vi "svl_Exp Avg Resampled Level Core (N Ch).vi"(0 "scaled signals":T1(array[cluster]) {"even angle signal" format="%.2f"; "dr" format="%.2f"; "r0" format="%.2f"}, 2 "sampling frequency [Hz]":dbl, 5 "filter coefficients (in)":T2 {"Forward Coefficients" format="%.2f"; "Reverse Coefficients" format="%.2f"}, 7 "initial values (impulse)":dbl[](array[numeric]) format="%.2f", 9 "init/cont (init:F)":bool, 11 "error in (no error)":errorcluster, 12 "initial values (exp)":dbl[](array[numeric]) format="%.2f", 13 "exponential mode":enum16{"Slow", "Fast", "Impulse", "Custom"}(ring)=enum."Fast") -> (4 "exp avg signals":T1(array[cluster]) {"even angle signal" format="%.2f"; "dr" format="%.2f"; "r0" format="%.2f"}, 6 "dup filter coefficients":T2 {"Forward Coefficients" format="%.2f"; "Reverse Coefficients" format="%.2f"}, 8 "final values (impulse)":dbl[](array[numeric]) format="%.2f", 14 "final values (exp)":dbl[](array[numeric]) format="%.2f", 15 "error out":errorcluster)   [LabVIEW 2017]
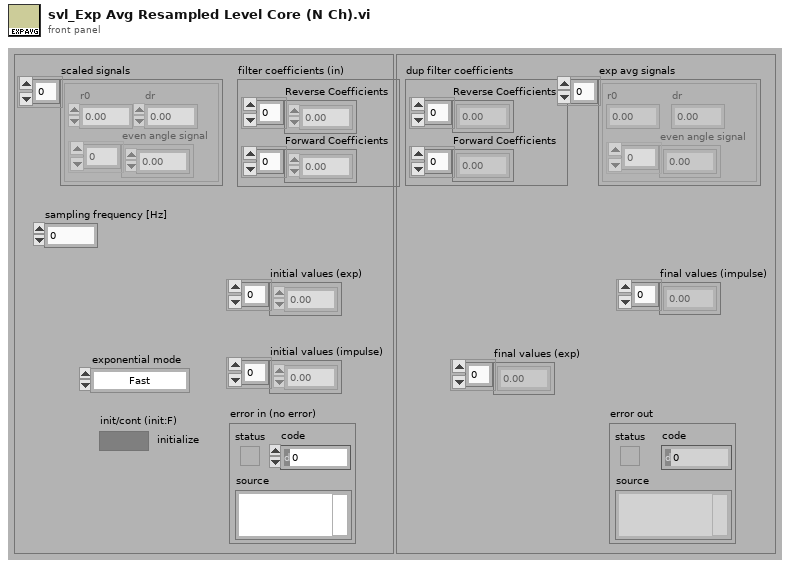
[diagram p1: front panel]
types:
  T1 = cluster{"r0":dbl, "dr":dbl, "even angle signal":dbl[]}[]
  T2 = cluster{"Reverse Coefficients":dbl[], "Forward Coefficients":dbl[]}
  T3 = cluster{"r0":dbl, "dr":dbl, "even angle signal":dbl[]}
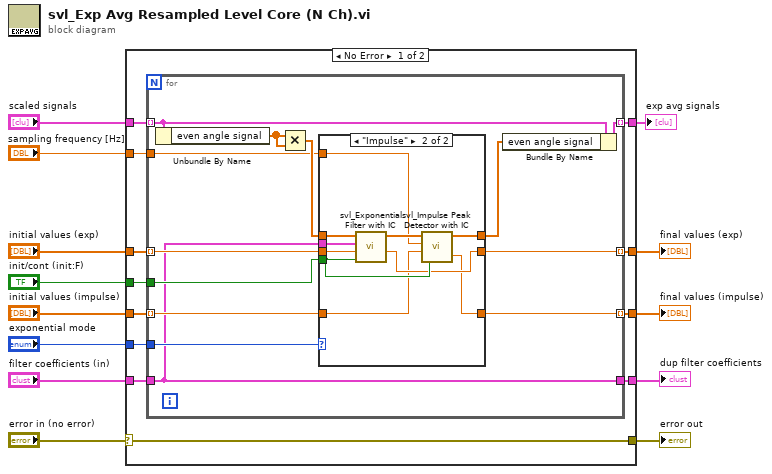
[diagram p0: block diagram]
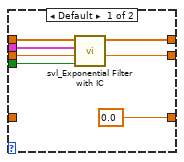
[diagram p2: hidden frame]
diagram:
  n1 = case shown="No Error" "error in (no error)" {
    selector: "error in (no error)" -> [w19 w57]
    tunnel: "initial values (exp)" -> [w25 w59]
    tunnel: "scaled signals" -> [w24 w56]
    tunnel: "exponential mode" -> [w23 _]
    tunnel: "filter coefficients (in)" -> [w22 w58]
    tunnel: "init/cont (init:F)" -> [w21 _]
    tunnel: [w20 w59] -> w8
    tunnel: [w19 w57] -> w7
    tunnel: "initial values (impulse)" -> [w18 w60]
    tunnel: [w17 w60] -> w5
    tunnel: [w16 w58] -> w4
    tunnel: "sampling frequency [Hz]" -> [w15 _]
    tunnel: [w14 w56] -> w1
    frame No Error {
      n2 = for {
        tunnel: w24 -> [w29] mode=indexing
        tunnel: w25 -> [w36] mode=indexing
        tunnel: w23 -> [w38]
        tunnel: w22 -> [w31]
        tunnel: w21 -> [w35]
        tunnel: [w34] -> w20 mode=indexing
        tunnel: w18 -> [w33] mode=indexing
        tunnel: [w32] -> w17 mode=indexing
        tunnel: [w31] -> w16
        tunnel: w15 -> [w30]
        tunnel: [w28] -> w14 mode=indexing
        n3 = Unbundle By Name(w29) -> ("even angle signal"=w26:dbl[])
        n4 = Multiply(x=w26, y=w26) -> (x*y=w37:dbl[])
        n5 = case shown="\"Impulse\"" w38 {
          tunnel: w37 -> [w45 w55]
          tunnel: w31 -> [w44 w54]
          tunnel: w36 -> [w43 w53]
          tunnel: w35 -> [w42 w51]
          tunnel: [w41 w50] -> w27
          tunnel: [w40 w49] -> w34
          tunnel: w33 -> [_ w48]
          tunnel: [0.0 ("final filter state") w47] -> w32
          tunnel: w30 -> [_ w46]
          frame Default {
            n6 = call <vilib>:"svl_Exponential Filter with IC.vi"("init/cont (init:F)"=w42, "initial filter state"=w43, "filter coefficients"=w44, "X"=w45) -> ("final filter state"=w40:dbl, "filtered X"=w41:dbl[])  [unwired: 5 in, 1 out]
          }
          frame "Impulse" {
            n7 = call <vilib>:"svl_Exponential Filter with IC.vi"("init/cont (init:F)"=w51, "initial filter state"=w53, "filter coefficients"=w54, "X"=w55) -> ("final filter state"=w49:dbl, "filtered X"=w52:dbl[])  [unwired: 5 in, 1 out]
            n8 = call <vilib>:"svl_Impulse Peak Detector with IC.vi"("init/cont (init:F)"=w51, "initial filter state"=w48, "sampling frequency [Hz]"=w46, "X"=w52) -> ("final filter state"=w47:dbl, "filtered X"=w50:dbl[])
          }
        }
        n9 = Bundle By Name(cluster=w29, "even angle signal"=w27) -> (w28:T3)
      }
    }
    frame Error {
    }
  }
  "dup filter coefficients" <- w4
  "final values (exp)" <- w8
  "error out" <- w7
  "final values (impulse)" <- w5
  "exp avg signals" <- w1
